vi "Str array to dbl array.vi"(8 "Error in (no error)":errorcluster, 11 "String array in":string="[1,23-2-3]\n[4-3,22-2]\n[3-4,01-8]\n[0-7-6,66]") -> (0 "Error out":errorcluster, 3 "Double array out":dbl[][](array[numeric]))   [LabVIEW 2012]
uses:
  <vilib>/regexp/Match Regular Expression.xnode
panel:
  # "String array to double array"
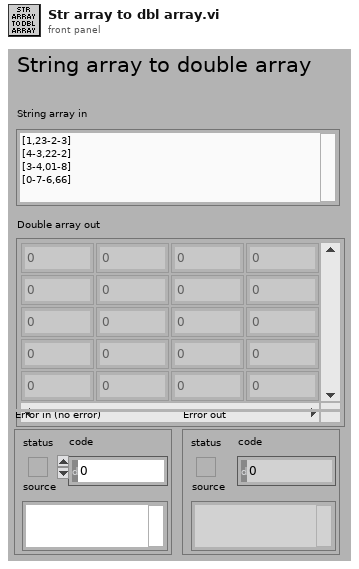
[diagram p1: front panel]
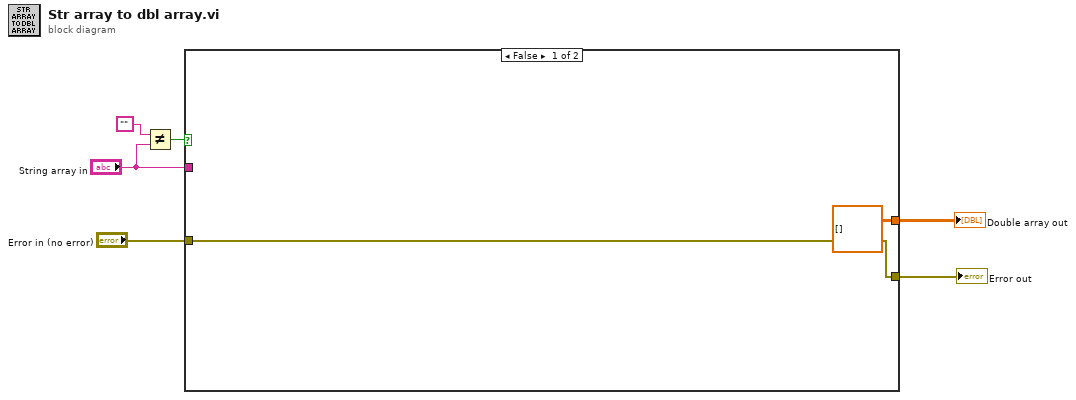
[diagram p0: block diagram]
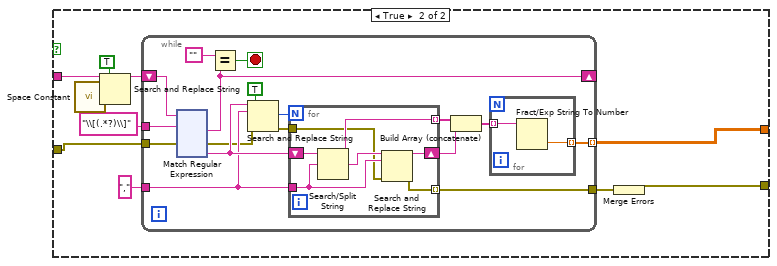
[diagram p2: hidden frame]
diagram:
  n1 = Not Equal?(x="", y="String array in") -> (x != y?=w3:bool)
  n2 = case shown="False" w3 {
    tunnel: "String array in" -> [_ w17]
    tunnel: [dbl[][] [] w13] -> w6
    tunnel: "Error in (no error)" -> [w7 w11]
    tunnel: [w7 w9] -> w4
    frame False {
    }
    frame True {
      n3 = call <vilib>:"Space Constant.vi"() -> ("String"=w18:string)
      n4 = Search and Replace String(replace all?=TRUE ("replace all? (F)"), input string=w17, search string=w18) -> (result string=w15:string)  [unwired: 5 in, 3 out]
      n5 = while {
        tunnel: "\\[(.*?)\\]" ("Regular expression") -> [w34]
        tunnel: [w29] -> w13 mode=indexing
        tunnel: "," ("Delimiter") -> [w26]
        shift-right: [w23] -> _
        shift-left: w15 -> [w35]
        tunnel: w11 -> [w21]
        tunnel: [w19] -> w10
        stop <- w25 stop-if-true
        n6 = xnode "Match Regular Expression"("input string"=w35, "regular expression"=w34, "error in"=w21) -> ("after match"=w23:string, "error out"=w22:errorcluster, "submatch 1"=w27:string)  [unwired: 3 in, 3 out]
        n7 = Equal?(x="", y=w23) -> (x = y?=w25:bool)
        n8 = Search and Replace String(replace all?=TRUE ("replace all? (F)"), input string=w27, search string=w26, error in=w22) -> (number of replacements=w33:i32, error out=w20:errorcluster)  [unwired: 4 in, 2 out]
        n9 = for {
          N: w33 -> [_]
          tunnel: [w44] -> w31 mode=indexing
          tunnel: w26 -> [w40]
          shift-right: [w41] -> w28
          shift-left: w27 -> [w43]
          tunnel: w20 -> [w39]
          tunnel: [w38] -> w19 mode=indexing
          n10 = Search/Split String(string=w43, search string/char (-)=w40) -> (substring before match=w44:string, match + rest of string=w42:string)  [unwired: 1 in, 1 out]
          n11 = Search and Replace String(input string=w42, search string=w40, error in=w39) -> (result string=w41:string, error out=w38:errorcluster)  [unwired: 5 in, 2 out]
        }
        n12 = Build Array (concatenate)(w31, w28) -> (w30:string[])
        n13 = for {
          tunnel: w30 -> [w37] mode=indexing
          tunnel: [w36] -> w29 mode=indexing
          n14 = Fract/Exp String To Number(string=w37) -> (number=w36:dbl)  [unwired: 3 in, 1 out]
        }
      }
      n15 = Merge Errors(w10) -> (w9:errorcluster)
    }
  }
  "Double array out" <- w6
  "Error out" <- w4
